vi "MS SQL_Set_Target_Done.vi"(8 "error in (no error)":errorcluster, 10 "Serial No":i32, 11 "Ref in":T1={"MS SQL Connection"=refnum, "UDL File"=path "", "Time"="", "DCODE"="", "WIP+1"=0, "MC No?"=0, "POKAYOKE?"=FALSE, "Expected Result"="", "Result [Status]"="", "Clock"=0.0, "RFID"="", "WIP Queue"=refnum, "TS Parameter"={"ProfitCenterCode"="", "LineCode"="", "WorkOrderNumber"="", "Model"="", "Model_with_Prefix"="", "VendorCode"="", "SetParameterDateCode"="", "PokaYoke"=0, "Target"=1, "Live_DateCode"="", "CustomerPartNumber"="", "Hand"="", "sBarcode"=FALSE, "FCA"=0, "Ent_Stamp"=timestamp(0 s since 1904-01-01), "STS_CD"=0.0}, "Data_Queue"=[], "RFID Serial No."=""} {"TS Parameter"."FCA" format="%01d"; "TS Parameter"."Target" min=1 max=100000; "TS Parameter"."PokaYoke" min=0 max=1}) -> (0 "error out":errorcluster, 3 "Ref Out":T1={"MS SQL Connection"=refnum, "UDL File"=path "", "Time"="", "DCODE"="", "WIP+1"=0, "MC No?"=0, "POKAYOKE?"=FALSE, "Expected Result"="", "Result [Status]"="", "Clock"=0.0, "RFID"="", "WIP Queue"=refnum, "TS Parameter"={"ProfitCenterCode"="", "LineCode"="", "WorkOrderNumber"="", "Model"="", "Model_with_Prefix"="", "VendorCode"="", "SetParameterDateCode"="", "PokaYoke"=0, "Target"=1, "Live_DateCode"="", "CustomerPartNumber"="", "Hand"="", "sBarcode"=FALSE, "FCA"=0, "Ent_Stamp"=timestamp(0 s since 1904-01-01), "STS_CD"=0.0}, "Data_Queue"=[], "RFID Serial No."=""} {"TS Parameter"."FCA" format="%01d"; "TS Parameter"."Target" min=1 max=100000; "TS Parameter"."PokaYoke" min=0 max=1}, 4 "Target?":bool)   [LabVIEW 2020]
uses:
  Controls/TD SQL.ctl
  <vilib>/addons/database/Connection.llb/Conn ObjectReference.ctl
  Controls/WIP_State.ctl
  Controls/TS_Parameter.ctl
  MS_Global.vi
  <vilib>/addons/database/NI_Database_API.lvlib
panel:
  out "resulting string":string
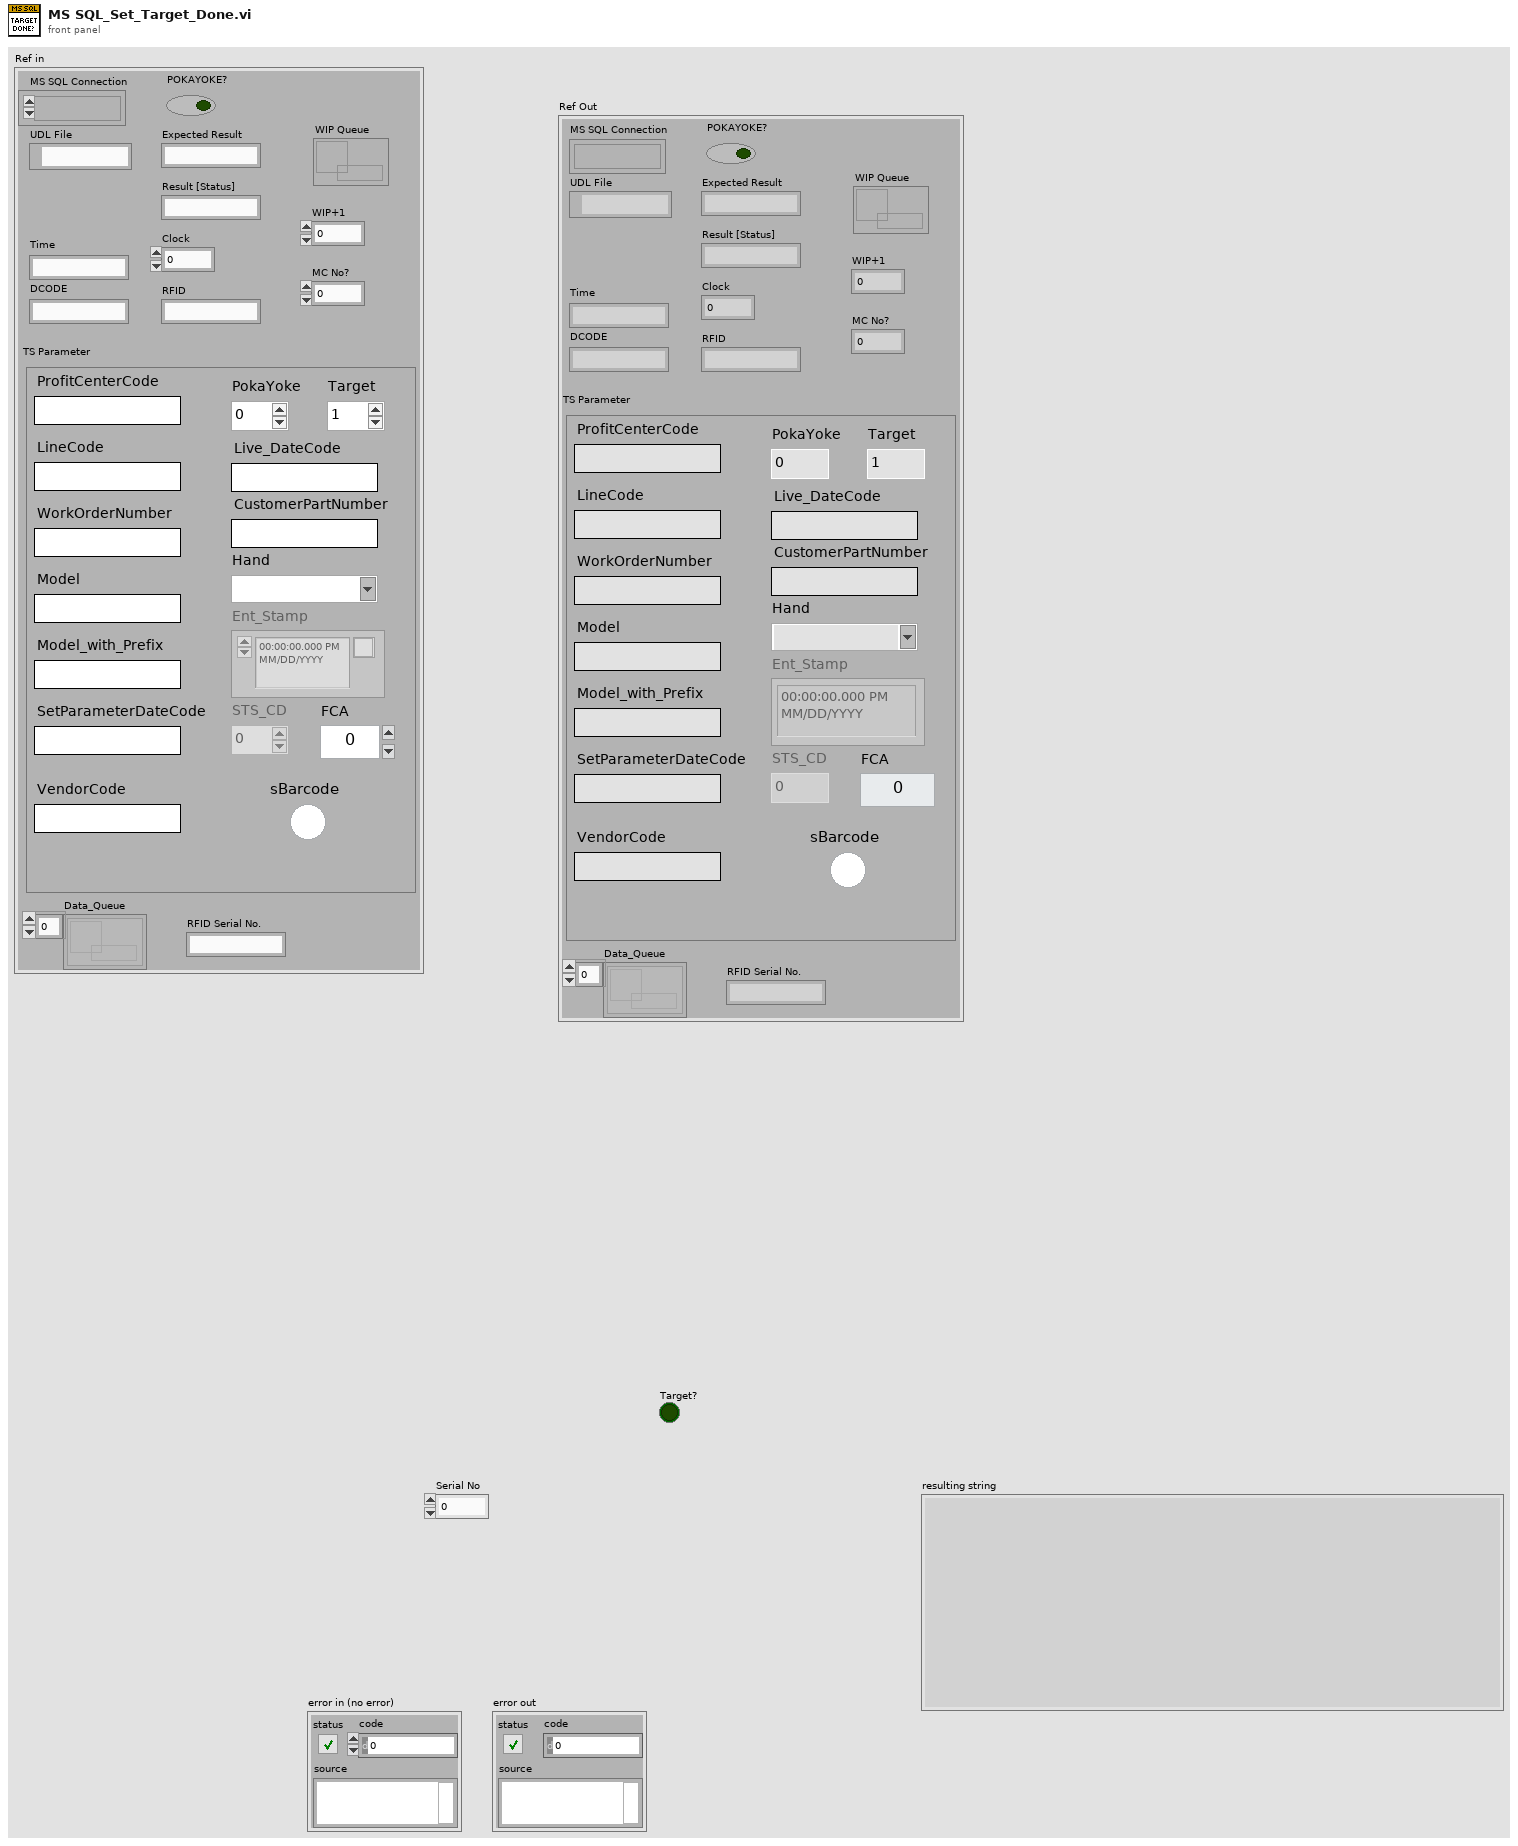
[diagram p1: front panel]
types:
  T1 = typedef "TD SQL.ctl" = cluster{"MS SQL Connection":T2, "UDL File":path, "Time":string, "DCODE":string, "WIP+1":i64, "MC No?":i32, "POKAYOKE?":bool, "Expected Result":string, "Result [Status]":string, "Clock":dbl, "RFID":string, "WIP Queue":refnum<queue>, "TS Parameter":T3, "Data_Queue":refnum<queue>[], "RFID Serial No.":string}
  T2 = typedef "NI_Database_API.lvlib/Conn ObjectReference.ctl" = refnum<k1>
  T3 = typedef "TS_Parameter.ctl" = cluster{"ProfitCenterCode":string, "LineCode":string, "WorkOrderNumber":string, "Model":string, "Model_with_Prefix":string, "VendorCode":string, "SetParameterDateCode":string, "PokaYoke":i32, "Target":i32, "Live_DateCode":string, "CustomerPartNumber":string, "Hand":string, "sBarcode":bool, "FCA":i32, "Ent_Stamp":timestamp, "STS_CD":dbl}
  T4 = typedef "WIP_State.ctl" = enum16{"Open", "Read", "Write", "Read WIP", "Flush", "Close"}
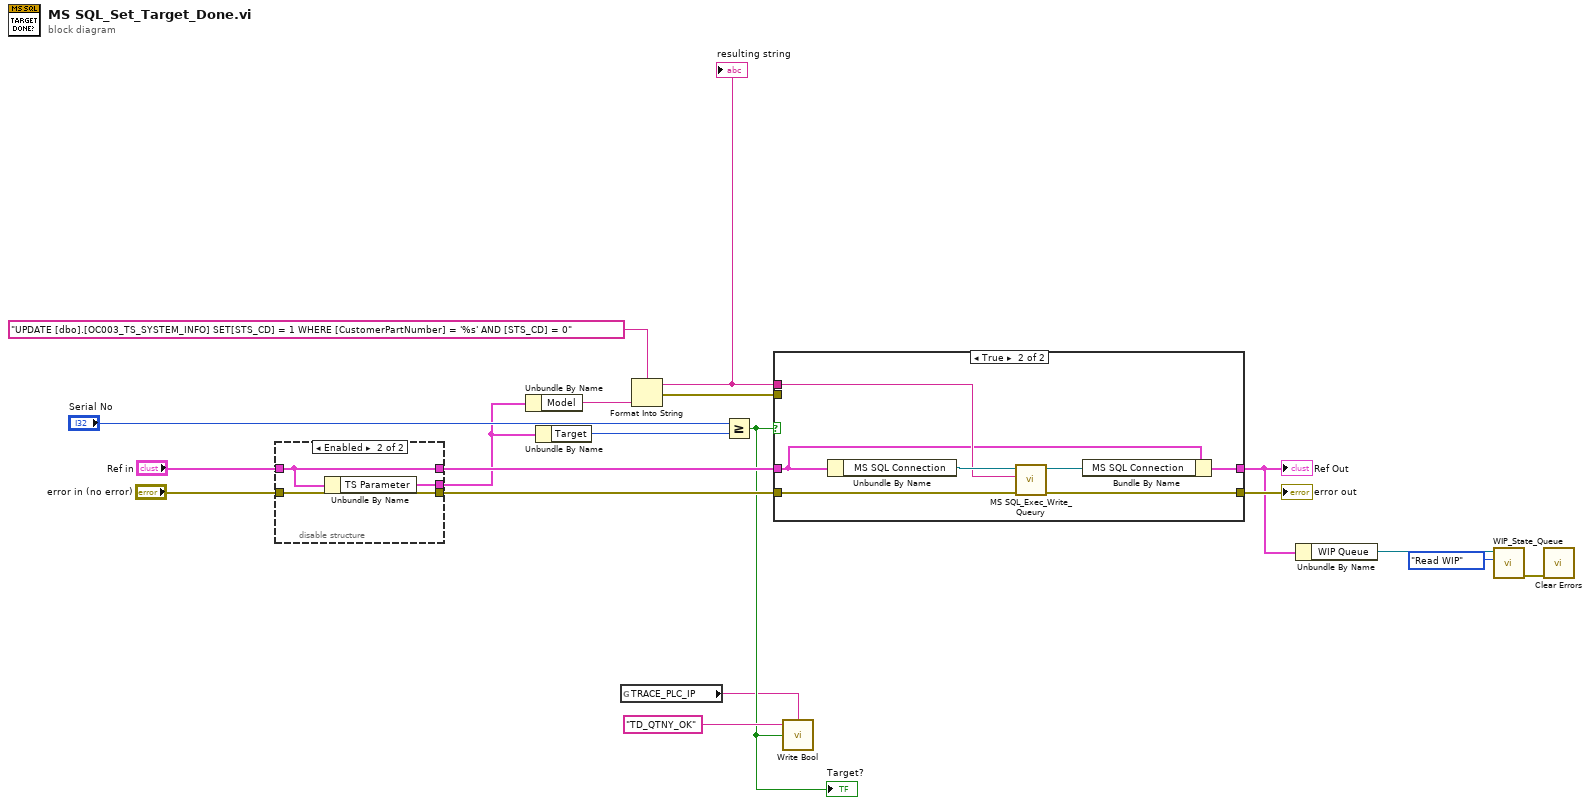
[diagram p0: block diagram]
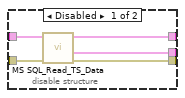
[diagram p2: hidden frame]
diagram:
  n1 = disable-structure shown="Enabled" {
    disable-tunnel: "Ref in" -> [w24 w26]
    disable-tunnel: "error in (no error)" -> [w23 w27]
    disable-tunnel: [w22 w27] -> w16
    disable-tunnel: [w21 w26] -> w14
    disable-tunnel: [w20 w25] -> w2
    frame Disabled {
      n2 = call "MS SQL_Read_TS_Data.vi"("error in (no error)"=w23, "Ref in"=w24) -> ("error out"=w22:errorcluster, "TS Parameter"=w20:T3, "Ref Out"=w21:T1)  [unwired: 2 in, 5 out]
    }
    frame Enabled {
      n3 = Unbundle By Name(w26) -> ("TS Parameter"=w25:T3)
    }
  }
  n4 = Unbundle By Name(w2) -> ("Model"=w1:string)
  n5 = Unbundle By Name(w2) -> ("Target"=w3:i32)
  n6 = global read "MS_Global.vi" "TRACE_PLC_IP"() -> (w8:string)
  n7 = Format Into String(format string="UPDATE [dbo].[OC003_TS_SYSTEM_INFO] SET[STS_CD] = 1 WHERE [CustomerPartNumber] = '%s' AND [STS_CD] = 0" ("Query"), w1) -> (resulting string=w11:string, error out=w12:errorcluster)  [unwired: 2 in]
  "resulting string" <- w11
  n8 = Greater Or Equal?(x="Serial No", y=w3) -> (x >= y?=w9:bool)
  "Target?" <- w9
  n9 = case shown="True" w9 {
    tunnel: w16 -> [w28 w30]
    tunnel: w11 -> [_ w35]
    tunnel: w14 -> [w29 w33]
    tunnel: [w28 w32] -> w13
    tunnel: [w29 w31] -> w5
    tunnel: w12 -> [_ _]
    frame False {
    }
    frame True {
      n10 = Unbundle By Name(w33) -> ("MS SQL Connection"=w36:T2)
      n11 = call "MS SQL_Exec_Write_Queury.vi"("error in (no error)"=w30, "Query"=w35, "Refnum in"=w36) -> ("error out"=w32:errorcluster, "Refnum out"=w34:T2)  [unwired: 7 in]
      n12 = Bundle By Name(cluster=w33, "MS SQL Connection"=w34) -> (w31:T1)
    }
  }
  "Ref Out" <- w5
  "error out" <- w13
  n13 = call "Write Bool.vi"("Network Path"=w8, "Int"=w9, "Tag Name"="TD_QTNY_OK" ("Network Path")) -> ()  [unwired: 2 in]
  n14 = Unbundle By Name(w5) -> ("WIP Queue"=w6:refnum<queue>)
  n15 = call "WIP_State_Queue.vi"("State In"=WIP_State."Read WIP", "Queue In"=w6) -> ("error out"=w4:errorcluster)  [unwired: 7 in, 2 out]
  n16 = call <vilib>:"Clear Errors.vi"("error in (no error)"=w4) -> ()  [unwired: 5 in, 2 out]
